vi "Teleop.vi"(10 "Match Info":T1={"Autonomous Elapsed Seconds"=0.0, "TeleOp Elapsed Seconds"=0.0, "Disabled Elapsed Seconds"=0.0, "Visited Autonomous"=FALSE, "Visited TeleOp"=FALSE, "Visited Disabled"=FALSE, "Autonomous Settings"={"Autonomous Style"=enum."Independent", "VI Refnum"=refnum}}, 11 "Call Context":T2) -> ()   [LabVIEW 2013]
doc: "This VI is called for each TeleOp packet received from the DS where the robot is not disabled. It is often used to read from the joysticks and update I/O or to update setpoints for timed control loops. It should complete and return within 20 milliseconds or it may miss DS packets."
uses:
  <vilib>/Rock Robotics/WPI/DriverStation/WPI_DriverStationDerivedRobotMode.ctl
  <vilib>/Rock Robotics/WPI/DriverStation/WPI_DriverStationMatch Info.ctl
  <vilib>/Rock Robotics/WPI/Relay/WPI_RelayValue.ctl
  Robot Global Data.vi
  <vilib>/Rock Robotics/WPI/Joystick/WPI_JoystickGetSetRefNum.vi
  <vilib>/Rock Robotics/WPI/Compressor/WPI_CompressorGetSetRefNum.vi
panel:
  in  "Release to Retract":u32=3000
  in  "Time Between Open and Shoot":u32=2000
  in  "GO BUTTON?":bool=TRUE
  out "Numeric 1":dbl(slide) scale=0.0..100.0
  out "Boolean 2":bool
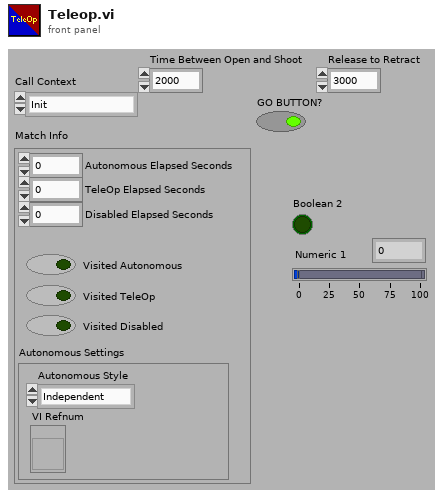
[diagram p1: front panel]
types:
  T1 = typedef "WPI_DriverStationMatch Info.ctl" = cluster{"Autonomous Elapsed Seconds":dbl, "TeleOp Elapsed Seconds":dbl, "Disabled Elapsed Seconds":dbl, "Visited Autonomous":bool, "Visited TeleOp":bool, "Visited Disabled":bool, "Autonomous Settings":cluster{"Autonomous Style":enum16{"Iterative", "Independent"}, "VI Refnum":refnum<vi>}}
  T2 = typedef "WPI_DriverStationDerivedRobotMode.ctl" = enum16{"Init", "Execute", "Stop"}
  T3 = typedef "WPI_RelayValue.ctl" = enum16{"Off", "On", "Forward", "Reverse"}
  T4 = typedef "WPI_JoystickDevRef.ctl" = cluster{"Device":T5}
  T5 = typedef "WPI_JoystickDeviceEnum.ctl" = enum16{"USB 1", "USB 2", "USB 3", "USB 4", "Kinect 1", "Kinect 2"}
  T6 = typedef "WPI_JoystickButtonState.ctl" = cluster{"Button 1":bool, "Button 2":bool, "Button 3":bool, "Button 4":bool, "Button 5":bool, "Button 6":bool, "Button 7":bool, "Button 8":bool, "Button 9":bool, "Button 10":bool, "Button 11":bool, "Button 12":bool}
  T7 = cluster{"axis 1 (x)":dbl, "axis 2 (y)":dbl, "axis 3 (throttle)":dbl, "axis 4":dbl, "axis 5":dbl, "axis 6":dbl}
  T8 = typedef "WPI_RelayDevRef.ctl" = cluster{"DevStatus":errorcluster, "Relay Channel":T9, "Digital Module":T10, "Relay Direction":T11}
  T9 = typedef "FPGA_DIORelayChannel.ctl" = enum8{"Relay 1", "Relay 2", "Relay 3", "Relay 4", "Relay 5", "Relay 6", "Relay 7", "Relay 8", "Invalid"}
  T10 = typedef "FPGA_TypedefDigitalModule.ctl" = enum16{"Digital Module 1", "Digital Module 2"}
  T11 = typedef "WPI_RelayDirection.ctl" = enum16{"Both directions", "Forward only", "Reverse only"}
  T12 = typedef "WPI_CompressorDevRef.ctl" = cluster{"DevStatus":errorcluster, "DigitalInputDevRef":T13, "RelayDevRef":T8}
  T13 = typedef "WPI_DigitalInputDevRef.ctl" = cluster{"DevStatus":errorcluster, "DIO Channel":T14, "Digital Module":T10}
  T14 = typedef "FPGA_DIOChannel.ctl" = enum8{"DIO 1", "DIO 2", "DIO 3", "DIO 4", "DIO 5", "DIO 6", "DIO 7", "DIO 8", "DIO 9", "DIO 10", "DIO 11", "DIO 12", "DIO 13", "DIO 14", "Invalid"}
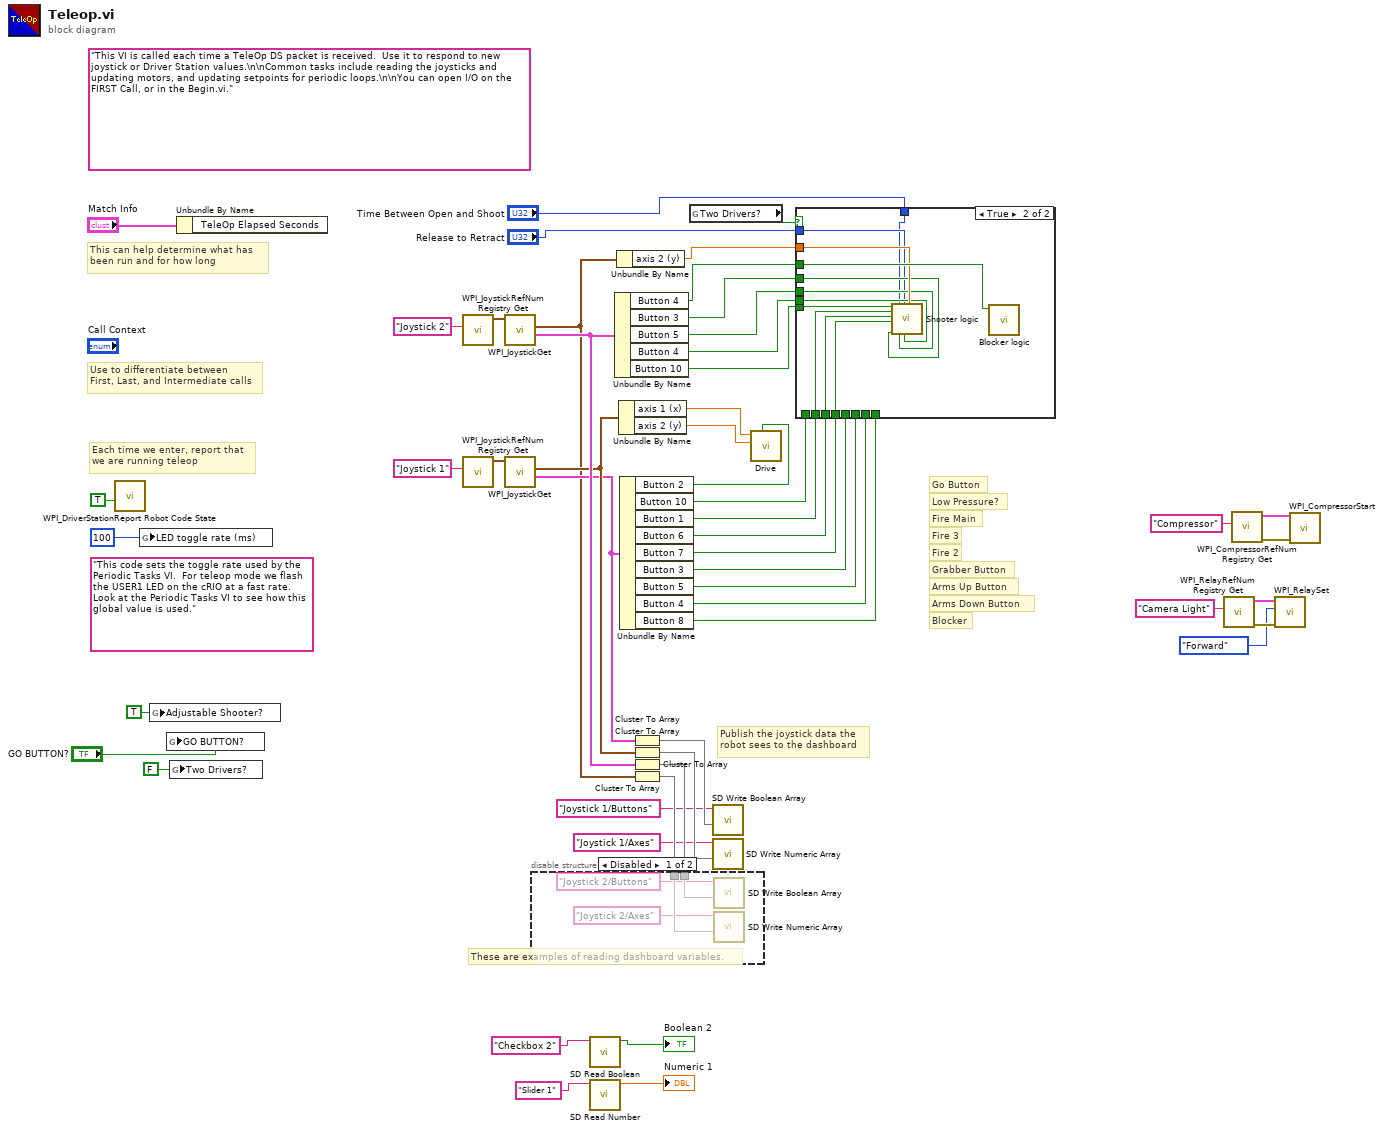
[diagram p0: block diagram]
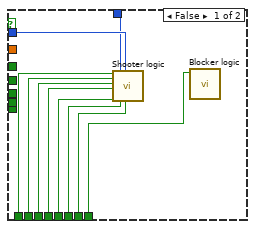
[diagram p2: hidden frame]
diagram:
  (unwired) "This code sets the toggle rate used by the Periodic Tasks VI.  For teleop mode we flash the USER1 LED on the cRIO at a fast rate.  Look at the Periodic Tasks VI to see how this global value is used."
  (unwired) "This VI is called each time a TeleOp DS packet is received.  Use it to respond to new joystick or Driver Station values.\n\nCommon tasks include reading the joysticks and updating motors, and updating setpoints for periodic loops.\n\nYou can open I/O on the FIRST Call, or in the Begin.vi."
  # "Blocker"
  # "Go Button"
  # "Arms Up Button"
  # "Arms Down Button"
  # "Grabber Button"
  # "Fire 2"
  # "Fire 3"
  # "Fire Main"
  # "Low Pressure?"
  # "These are examples of reading dashboard variables."
  # "Publish the joystick data the\nrobot sees to the dashboard"
  # "Each time we enter, report that\nwe are running teleop"
  # "Use to differentiate between\nFirst, Last, and Intermediate calls"
  # "This can help determine what has\nbeen run and for how long"
  n1 = call <vilib>:"WPI_DriverStationReport Robot Code State.vi"("TeleOp"=TRUE ("Autonomous")) -> ()  [unwired: 10 in, 1 out]
  n2 = global write "Robot Global Data.vi" "LED toggle rate (ms)"(u32 100 ("LED ms toggle rate")) -> ()
  n3 = global write "Robot Global Data.vi" "Adjustable Shooter?"(TRUE ("GO BUTTON?")) -> ()
  n4 = global write "Robot Global Data.vi" "GO BUTTON?"("GO BUTTON?") -> ()
  n5 = global write "Robot Global Data.vi" "Two Drivers?"(FALSE ("GO BUTTON?")) -> ()
  n6 = Unbundle By Name("Match Info") -> ()  [unwired: 1 out]
  n7 = call <vilib>:"WPI_JoystickRefNum Registry Get.vi"("refnum name"="Joystick 2") -> ("JoystickDevRef"=w38:T4)  [unwired: 1 in, 9 out]
  n8 = call <vilib>:"WPI_JoystickRefNum Registry Get.vi"("refnum name"="Joystick 1") -> ("JoystickDevRef"=w49:T4)  [unwired: 1 in, 9 out]
  n9 = call <vilib>:"WPI_JoystickGet.vi"("JoystickDevRef"=w38) -> ("Buttons"=w35:T6, "Axes"=w5:T7)  [unwired: 1 in, 4 out]
  n10 = call <vilib>:"WPI_JoystickGet.vi"("JoystickDevRef"=w49) -> ("Buttons"=w32:T6, "Axes"=w33:T7)  [unwired: 1 in, 4 out]
  n11 = call <vilib>:"SD Read Boolean.vi"("Name"="Checkbox 2" ("refnum name")) -> ("Boolean"=→"Boolean 2":bool)  [unwired: 8 in, 2 out]
  n12 = call <vilib>:"SD Read Number.vi"("Name"="Slider 1" ("refnum name")) -> ("Numeric"=→"Numeric 1":dbl)  [unwired: 8 in, 2 out]
  n13 = Unbundle By Name(w35) -> ("Button 4"=w10:bool, "Button 3"=w13:bool, "Button 5"=w12:bool, "Button 4"=w2:bool, "Button 10"=w3:bool)
  n14 = Unbundle By Name(w5) -> ("axis 2 (y)"=w4:dbl)
  n15 = Unbundle By Name(w33) -> ("axis 1 (x)"=w43:dbl, "axis 2 (y)"=w44:dbl)
  n16 = Unbundle By Name(w32) -> ("Button 2"=w22:bool, "Button 10"=w19:bool, "Button 1"=w18:bool, "Button 6"=w17:bool, "Button 7"=w16:bool, "Button 3"=w15:bool, "Button 5"=w14:bool, "Button 4"=w11:bool, "Button 8"=w1:bool)
  n17 = Cluster To Array(cluster=w32) -> (array=w46:bool[])
  n18 = Cluster To Array(cluster=w33) -> (array=w45:dbl[])
  n19 = Cluster To Array(cluster=w35) -> (array=w34:bool[])
  n20 = Cluster To Array(cluster=w5) -> (array=w36:dbl[])
  n21 = disable-structure shown="Disabled" {
    disable-tunnel: w36 -> [w55 _]
    disable-tunnel: w34 -> [w54 _]
    frame Disabled {
      n22 = call <vilib>:"SD Write Boolean Array.vi"("Boolean Array"=w54, "Name"="Joystick 2/Buttons") -> ()  [unwired: 8 in, 2 out]
      n23 = call <vilib>:"SD Write Numeric Array.vi"("Numeric Array"=w55, "Name"="Joystick 2/Axes") -> ()  [unwired: 8 in, 2 out]
    }
    frame Enabled {
    }
  }
  n24 = global read "Robot Global Data.vi" "Two Drivers?"() -> (w24:bool)
  n25 = call <vilib>:"SD Write Boolean Array.vi"("Boolean Array"=w46, "Name"="Joystick 1/Buttons") -> ()  [unwired: 8 in, 2 out]
  n26 = call <vilib>:"SD Write Numeric Array.vi"("Numeric Array"=w45, "Name"="Joystick 1/Axes") -> ()  [unwired: 8 in, 2 out]
  n27 = call "Drive.vi"("GO BUTTON"=w22, "Y axis value"=w44, "X axis value"=w43) -> ()  [unwired: 9 in]
  n28 = case shown="True" w24 {
    tunnel: "Time Between Open and Shoot" -> [w56 w66]
    tunnel: "Release to Retract" -> [w57 w67]
    tunnel: w19 -> [w65 _]
    tunnel: w18 -> [w64 w76]
    tunnel: w17 -> [w63 w75]
    tunnel: w16 -> [w62 w74]
    tunnel: w15 -> [w60 _]
    tunnel: w14 -> [w61 _]
    tunnel: w12 -> [_ w70]
    tunnel: w13 -> [_ w68]
    tunnel: w3 -> [_ w73]
    tunnel: w11 -> [w59 _]
    tunnel: w10 -> [_ w72]
    tunnel: w4 -> [_ w71]
    tunnel: w2 -> [_ w69]
    tunnel: w1 -> [w58 _]
    frame False {
      n29 = call "Shooter logic.vi"("Low Pressure?"=w65, "Fire Main"=w64, "Fire 3"=w63, "Fire 2"=w62, "Grabber Button"=w60, "Time Between Open and Shoot"=w56, "Arms Up button"=w61, "Release to Retract"=w57, "Arms Down Button"=w59) -> ()  [unwired: 11 in]
      n30 = call "Blocker logic.vi"("Botton on"=w58) -> ()  [unwired: 11 in]
    }
    frame True {
      n31 = call "Shooter logic.vi"("Low Pressure?"=w73, "Fire Main"=w76, "Fire 3"=w75, "Fire 2"=w74, "Grabber Button"=w68, "Time Between Open and Shoot"=w66, "Arms Up button"=w70, "Release to Retract"=w67, "Arms Down Button"=w69, "Arms up and down"=w71) -> ()  [unwired: 10 in]
      n32 = call "Blocker logic.vi"("Botton on"=w72) -> ()  [unwired: 11 in]
    }
  }
  n33 = call <vilib>:"WPI_RelayRefNum Registry Get.vi"("refnum name"="Camera Light") -> ("error out"=w28:errorcluster, "RelayDevRef"=w27:T8)  [unwired: 9 in]
  n34 = call <vilib>:"WPI_CompressorRefNum Registry Get.vi"("refnum name"="Compressor") -> ("error out"=w42:errorcluster, "CompressorDevRef"=w41:T12)  [unwired: 9 in]
  n35 = call <vilib>:"WPI_RelaySet.vi"("error in (no error)"=w28, "RelayValue"=WPI_RelayValue."Forward", "RelayDevRef"=w27) -> ()  [unwired: 7 in, 2 out]
  n36 = call <vilib>:"WPI_CompressorStart.vi"("error in (no error)"=w42, "CompressorDevRef"=w41) -> ()  [unwired: 8 in, 2 out]
